vi "2.vi"() -> ()   [LabVIEW 2021]
panel:
  out "sum":u64
  out "Array":u64[](array[numeric])
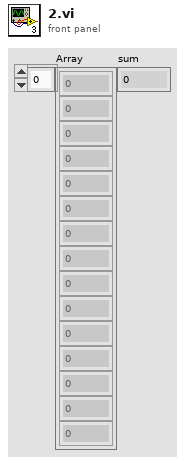
[diagram p1: front panel]
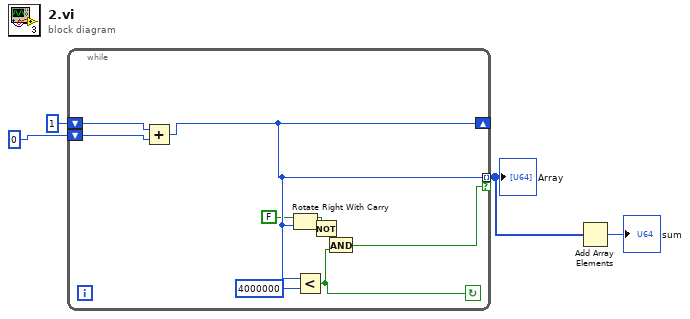
[diagram p0: block diagram]
diagram:
  n1 = while {
    shift-right: [w9] -> _
    shift-left: u64 1 -> [w13]
    shift-left: u64 0 -> [w12]
    tunnel: [w9] -> w2 mode=indexing if=w6
    stop <- w10 continue-if-true
    n2 = Add(x=w13, y=w12) -> (x+y=w9:u64)
    n3 = Rotate Right With Carry(2:w9, 3:FALSE ("carry")) -> (1:w7:bool)  [unwired: 1 out]
    n4 = Less?(x=w9, y=u64 4000000) -> (x < y?=w10:bool)
    n5 = Not(x=w7) -> (.not. x?=w5:bool)
    n6 = And(x=w5, y=w10) -> (x .and. y?=w6:bool)
  }
  "Array" <- w2
  n7 = Add Array Elements(numeric array=w2) -> (sum=→"sum":u64)
